vi "spin_diode_effect_test.vi"() -> ()   [LabVIEW 2017]
uses:
  <userlib>/niRF/niQuickSyn/Core/Properties/RF Frequency/PropertyType.ctl
  <userlib>/niRF/niQuickSyn/Core/Properties/RF Power/PropertyType.ctl
  <userlib>/niRF/niQuickSyn/Core/Properties/AM State/PropertyType.ctl
  <userlib>/niRF/niQuickSyn/Core/Properties/FM Sensitivity/PropertyType.ctl
  <userlib>/niRF/niQuickSyn/Core/Properties/VISA Handle/PropertyType.ctl
  <vilib>/Utility/error.llb/DialogType.ctl
  <userlib>/niRF/niQuickSyn/Core/Properties/RF Output/PropertyType.ctl
  <vilib>/DAQmx/write.llb/DAQmx Write (Analog Wfm 1Chan NSamp).vi
  <vilib>/DAQmx/read.llb/DAQmx Read (Analog 1D DBL 1Chan NSamp).vi
  <vilib>/DAQmx/create/channels.llb/DAQmx Create Channel (AO-Voltage-Basic).vi
  <vilib>/DAQmx/configure/timing.llb/DAQmx Timing (Sample Clock).vi
  <vilib>/DAQmx/create/channels.llb/DAQmx Create Channel (AI-Voltage-Basic).vi
  <vilib>/DAQmx/configure/trigger.llb/DAQmx Start Trigger (None).vi
  <vilib>/DAQmx/miscellaneous.llb/DAQmx Fill In Error Info.vi
  <vilib>/Analysis/3filter.llb/Butterworth Filter (DBL).vi
  <userlib>/niRF/niQuickSyn/QuickSyn API.lvlib
  <userlib>/niRF/niQuickSyn/Core/Properties/VISA Handle/VISA Handle.lvclass
  <vilib>/measure/NI_MABase.lvlib
  <userlib>/niRF/niQuickSyn/Core/Properties/RF Output/RF Output.lvclass
  <resource>/objmgr/daqmx.rc
  <vilib>/Analysis/NI_AALBase.lvlib
  <userlib>/niRF/niQuickSyn/Core/Properties/RF Frequency/RF Frequency.lvclass
  <userlib>/niRF/niQuickSyn/Core/Properties/RF Power/RF Power.lvclass
  <userlib>/niRF/niQuickSyn/Core/Properties/AM State/AM State.lvclass
  <userlib>/niRF/niQuickSyn/Core/Properties/FM Sensitivity/FM Sensitivity.lvclass
panel:
  out "SpectrumGraph 3":cluster{dbl[], "data":dbl[]}(graph)
  in  "Number of steps":i32=1000 min=2 step=1
  in  "RF Frequency Stop, Hz":T1=6000000000.0 format="%#_9p"
  out "SpectrumGraph 2":cluster{dbl[], "data":dbl[]}(graph)
  out "Voltage/4":dbl
  in  "AM Depth":T2=100.0 format="%#_9p"
  in  "Amplitude Modulation":T3=enum."Enabled"
  in  "RF Output":bool=TRUE
  in  "error in (no error)":errorcluster
  out "AI.Max":dbl=2.0
  out "AI.Min":dbl=-2.0
  out "AO.Max":dbl=1.0
  out "AO.Min":dbl=-1.0
  out "SpectrumGraph":cluster{dbl[], "data":dbl[]}(graph)
  in  "stop":bool
  out "ms passed":u32=1
  in  "ms to wait":u32=1
  out "error out":errorcluster={"status"=FALSE, "code"=1073676293, "source"="VISA Read in AKIP_read.vi->AKIP_error_check.vi->AKIP_output_on_off.vi->spin_diode_effect_test.vi"}
  in  "AI max":dbl=10.0 format="%0.2f"
  in  "AO max":dbl=0.5 format="%0.2f"
  in  "RF Power, dB":T4=-10.0
  in  "RF Frequency Start, Hz":T1=500000000.0 format="%#_9p"
  in  "Modulation frequency, Hz":dbl=10000.0 format="%0.1p"
  in  "Modulation amplitude, V":dbl=0.5 format="%0.3f"
  in  "AI channel":tag="DAQ6363/ai4"
  in  "AO channel":tag="DAQ6363/ao0"
  in  "Field, Oe":dbl
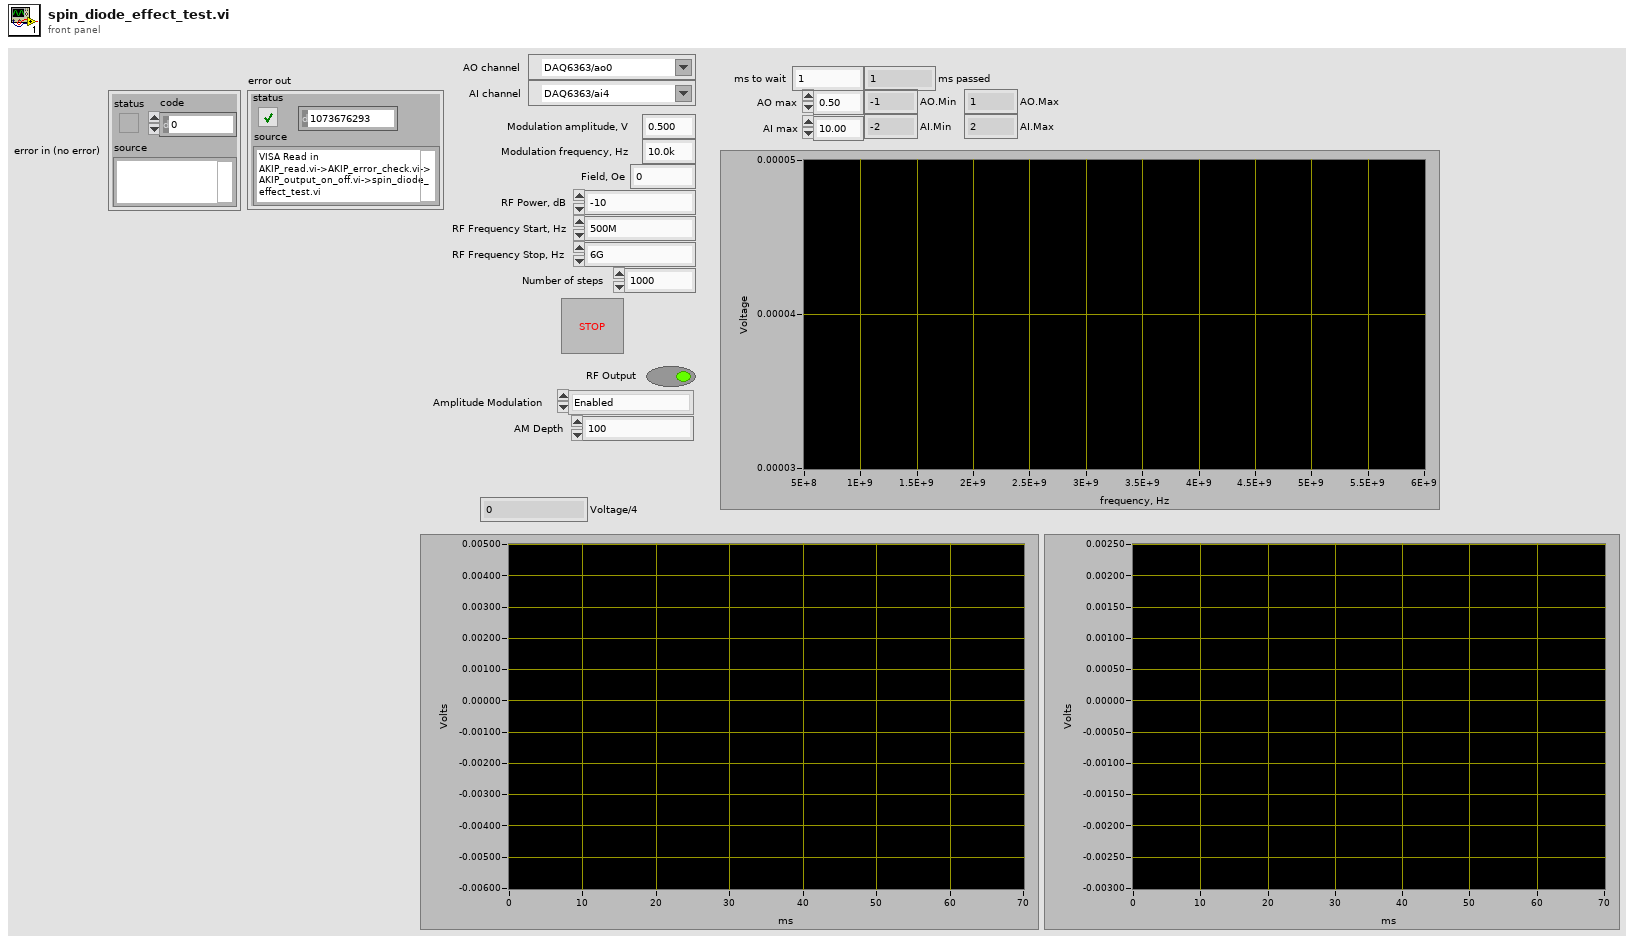
[diagram p1: front panel]
types:
  T1 = typedef "QuickSyn API.lvlib/RF Frequency.lvclass/PropertyType.ctl" = dbl
  T2 = typedef "QuickSyn API.lvlib/FM Sensitivity.lvclass/PropertyType.ctl" = dbl
  T3 = typedef "QuickSyn API.lvlib/AM State.lvclass/PropertyType.ctl" = enum16{"Disabled", "Enabled"}
  T4 = typedef "QuickSyn API.lvlib/RF Power.lvclass/PropertyType.ctl" = dbl
  T5 = enum16{"Sine Wave", "Triangle Wave", "Square Wave", "Sawtooth Wave"}
  T6 = typedef "QuickSyn API.lvlib/RF Output.lvclass/PropertyType.ctl" = bool
  T7 = typedef "DialogType.ctl" = u16
  T8 = typedef "QuickSyn API.lvlib/VISA Handle.lvclass/PropertyType.ctl" = refnum<visa-resource-name>
  T9 = typedef "QuickSyn API.lvlib/QuickSyn.lvclass/Session Handle.ctl" = refnum<data-value>
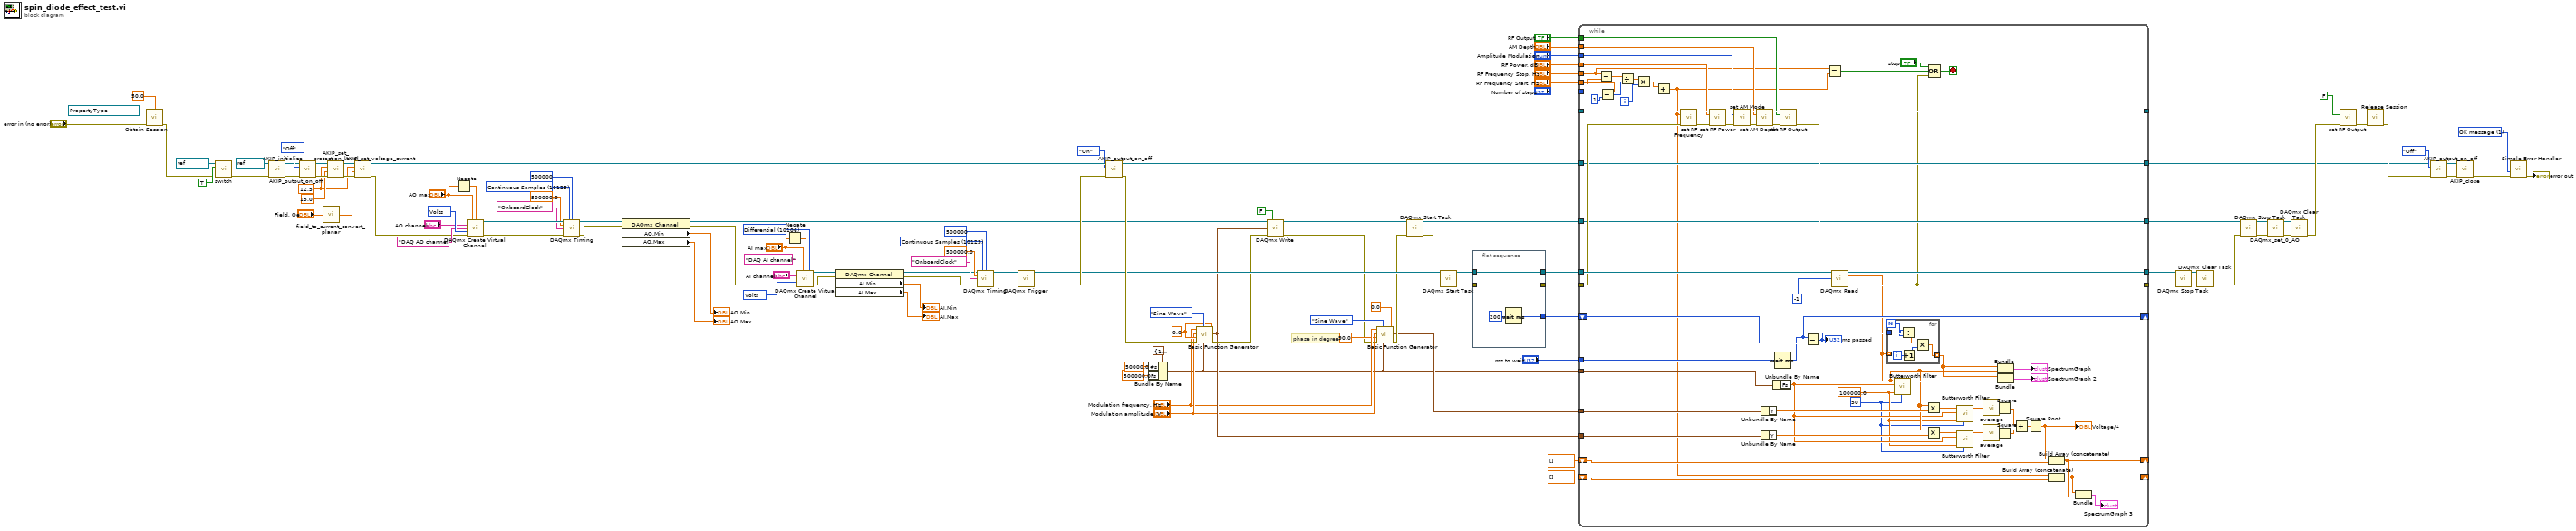
[diagram p0: block diagram]
diagram:
  w38 = 10123 items=["Finite Samples"=10178, "Continuous Samples"=10123, "Hardware Timed Single Point"=12522] ("sample mode")
  w76 = T7 1 items=["no dialog", "OK message", "continue or stop message", "OK message + warnings", "continue/stop + warnings"] ("type of dialog (OK msg:1)")
  w78 = 10348 items=["Volts"=10348, "From Custom Scale"=10065] ("units")
  w79 = 10106 items=["Default"=-1, "RSE"=10083, "NRSE"=10078, "Differential"=10106, "Pseudodifferential"=12529] ("input terminal configuration")
  w89 = 0.0 ("phase")
  w115 = 10123 items=["Finite Samples"=10178, "Continuous Samples"=10123, "Hardware Timed Single Point"=12522] ("sample mode")
  w116 = 10348 items=["Volts"=10348, "From Custom Scale"=10065] ("units")
  w101 = 12.5 ("Voltage")
  # "phase in degrees"
  n1 = call <userlib>:"Obtain Session.vi"("VISA resource name"=T8 "QuickSyn_generator", "Serial Timeout"=50.0, "error in (no error)"="error in (no error)") -> ("Session Handle"=w17:T9, "error out"=w28:errorcluster)  [unwired: 11 in]
  n2 = call "switch.vi"("error in (no error)"=w28, "Positive?"=TRUE, "Switch port (in)"=refnum<visa-resource-name> "Switch") -> ("error out"=w98:errorcluster)  [unwired: 7 in, 1 out]
  n3 = call "AKIP_initialize.vi"("error in (no error)"=w98, "VISA Refnum in"=refnum<visa-resource-name> "AKIP") -> ("error out"=w118:errorcluster, "VISA Refnum out"=w119:refnum<visa-resource-name>)  [unwired: 8 in]
  n4 = call "AKIP_output_on_off.vi"("error in (no error)"=w118, "Enum"=enum16{"On", "Off"}."Off", "VISA Refnum in"=w119) -> ("error out"=w105:errorcluster, "VISA Refnum out"=w104:refnum<visa-resource-name>)  [unwired: 7 in]
  n5 = call "field_to_current_convert_planar.vi"("Field, Oe"="Field, Oe") -> ("Current, A"=w1:dbl)
  n6 = call "AKIP_set_protection_level.vi"("error in (no error)"=w105, "Current Protection Level"=15.0, "Voltage Protection Level"=w101, "VISA resource name (in)"=w104) -> ("error out"=w102:errorcluster, "VISA resource name (out)"=w100:refnum<visa-resource-name>)  [unwired: 6 in]
  n7 = call "AKIP_set_voltage_current.vi"("error in (no error)"=w102, "Current"=w1, "Voltage"=w101, "VISA resource name (in)"=w100) -> ("error out"=w97:errorcluster, "VISA resource name (out)"=w88:refnum<visa-resource-name>)  [unwired: 6 in]
  n8 = Negate(x="AO max") -> (-x=w82:dbl)
  n9 = call-poly <vilib>:"DAQmx Create Virtual Channel.vi"("maximum value"="AO max", "minimum value"=w82, "physical channels"="AO channel", "name to assign"="DAQ AO channel", "units"=w116, "error in"=w97) -> ("task out"=w42:refnum<k21>, "error out"=w41:errorcluster)  [unwired: 8 in]
  n10 = call-poly <vilib>:"DAQmx Timing.vi"("task/channels in"=w42, "sample mode"=w38, "samples per channel"=500000, "rate"=500000.0, "source"=tag "OnboardClock", "error in"=w41) -> ("task out"=w39:refnum<k21>, "error out"=w40:errorcluster)  [unwired: 8 in]
  n11 = property class="DAQmx Channel"(reference=w39, error in=w40) -> (reference out=w65:refnum<k21>, error out=w64:errorcluster, "AO.Min"=→"AO.Min":dbl, "AO.Max"=→"AO.Max":dbl)
  n12 = Negate(x="AI max") -> (-x=w80:dbl)
  n13 = call-poly <vilib>:"DAQmx Create Virtual Channel.vi"("maximum value"="AI max", "minimum value"=w80, "input terminal configuration"=w79, "physical channels"="AI channel", "name to assign"="DAQ AI channel", "units"=w78, "error in"=w64) -> ("task out"=w61:refnum<k21>, "error out"=w59:errorcluster)  [unwired: 7 in]
  n14 = property class="DAQmx Channel"(reference=w61, error in=w59) -> (reference out=w60:refnum<k21>, error out=w58:errorcluster, "AI.Min"=→"AI.Min":dbl, "AI.Max"=→"AI.Max":dbl)
  n15 = call-poly <vilib>:"DAQmx Timing.vi"("task/channels in"=w60, "sample mode"=w115, "samples per channel"=500000, "rate"=500000.0, "source"=tag "OnboardClock", "error in"=w58) -> ("task out"=w113:refnum<k21>, "error out"=w112:errorcluster)  [unwired: 8 in]
  n16 = call-poly <vilib>:"DAQmx Trigger.vi"("task/channels in"=w113, "error in"=w112) -> ("task out"=w55:refnum<k21>, "error out"=w87:errorcluster)  [unwired: 12 in]
  n17 = call "AKIP_output_on_off.vi"("error in (no error)"=w87, "Enum"=enum16{"On", "Off"}."On", "VISA Refnum in"=w88) -> ("error out"=w85:errorcluster, "VISA Refnum out"=w15:refnum<visa-resource-name>)  [unwired: 7 in]
  n18 = Bundle By Name(cluster=cluster{"Fs":dbl, "#s":dbl} {"Fs"=1000.0, "#s"=1000.0} ("sampling info"), "#s"=50000.0, "Fs"=500000.0) -> (w19:cluster{"Fs":dbl, "#s":dbl})
  n19 = call <vilib>:"Basic Function Generator.vi"("offset"=w89, "sampling info"=w19, "signal type"=T5."Sine Wave", "error in (no error)"=w85, "phase"=w89, "amplitude"="Modulation amplitude, V", "frequency"="Modulation frequency, Hz") -> ("error out"=w29:errorcluster, "signal out"=w27:waveform(dbl))  [unwired: 2 in, 1 out]
  n20 = call-poly <vilib>:"DAQmx Write.vi"("task/channels in"=w65, "auto start"=FALSE, "data"=w27, "error in"=w29) -> ("task out"=w84:refnum<k21>, "error out"=w18:errorcluster)  [unwired: 9 in, 1 out]
  n21 = call <vilib>:"Basic Function Generator.vi"("offset"=0.0, "sampling info"=w19, "signal type"=T5."Sine Wave", "error in (no error)"=w18, "phase"=90.0, "amplitude"="Modulation amplitude, V", "frequency"="Modulation frequency, Hz") -> ("error out"=w21:errorcluster, "signal out"=w20:waveform(dbl))  [unwired: 2 in, 1 out]
  n22 = call <vilib>:"DAQmx Start Task.vi"("task/channels in"=w84, "error in"=w21) -> ("task out"=w13:refnum<k21>, "error out"=w54:errorcluster)  [unwired: 12 in]
  n23 = call <vilib>:"DAQmx Start Task.vi"("task/channels in"=w55, "error in"=w54) -> ("task out"=w67:refnum<k21>, "error out"=w66:errorcluster)  [unwired: 12 in]
  n24 = flat-sequence {
    tunnel: w66 -> [w124]
    tunnel: [w124] -> w72
    tunnel: w67 -> [w123]
    tunnel: [w123] -> w73
    tunnel: [w121] -> w69
    frame #0 {
      n25 = Wait (ms)(milliseconds to wait=u32 200) -> (millisecond timer value=w121:u32)
    }
  }
  n26 = while {
    tunnel: w73 -> [w190]
    tunnel: w72 -> [w160]
    tunnel: [w145] -> w71
    tunnel: [w189] -> w70
    shift-right: [w186] -> _
    shift-left: w69 -> [w187]
    tunnel: "ms to wait" -> [w188]
    tunnel: w27 -> [w185]
    tunnel: w20 -> [w184]
    tunnel: w19 -> [w174]
    tunnel: w17 -> [w162]
    tunnel: [w161] -> w16
    tunnel: w15 -> [w158]
    tunnel: [w158] -> w14
    tunnel: w13 -> [w157]
    tunnel: [w157] -> w12
    tunnel: "RF Output" -> [w156]
    tunnel: "AM Depth" -> [w155]
    tunnel: "Amplitude Modulation" -> [w154]
    tunnel: "RF Power, dB" -> [w153]
    tunnel: "Number of steps" -> [w151]
    tunnel: "RF Frequency Stop, Hz" -> [w142]
    tunnel: "RF Frequency Start, Hz" -> [w144]
    shift-right: [w137] -> _
    shift-left: dbl[] [] -> [w138]
    shift-right: [w134] -> _
    shift-left: T1[] [] -> [w135]
    i -> [w147]
    stop <- w140 stop-if-true
    w126 = 100000.0 ("low cutoff freq: fl")
    w125 = 50 ("order")
    n27 = Subtract(x=w142, y=w144) -> (x-y=w152:T1)
    n28 = Subtract(x=w151, y=1) -> (x-y=w149:i32)
    n29 = Divide(x=w152, y=w149) -> (x/y=w148:T1)
    n30 = Multiply(x=w148, y=w147) -> (x*y=w143:T1)
    n31 = Add(x=w143, y=w144) -> (x+y=w136:T1)
    n32 = call <userlib>:"set RF Frequency.vi"("Session Handle in"=w162, "RF Frequency, Hz (200M)"=w136, "error in (no error)"=w160) -> ("Session Handle out"=w165:T9, "error out"=w166:errorcluster)  [unwired: 11 in]
    n33 = call <userlib>:"set RF Power.vi"("Session Handle in"=w165, "RF Power, dB (0)"=w153, "error in (no error)"=w166) -> ("Session Handle out"=w168:T9, "error out"=w167:errorcluster)  [unwired: 11 in]
    n34 = call <userlib>:"set AM Mode.vi"("Session Handle in"=w168, "AM State"=w154, "error in (no error)"=w167) -> ("Session Handle out"=w163:T9, "error out"=w164:errorcluster)  [unwired: 11 in]
    n35 = call <userlib>:"set AM Depth.vi"("Session Handle in"=w163, "AM Depth"=w155, "error in (no error)"=w164) -> ("Session Handle out"=w169:T9, "error out"=w170:errorcluster)  [unwired: 11 in]
    n36 = Unbundle By Name(w184) -> ("Y"=w176:dbl[])
    n37 = Unbundle By Name(w185) -> ("Y"=w177:dbl[])
    n38 = Unbundle By Name(w174) -> ("Fs"=w127:dbl)
    n39 = Wait (ms)(milliseconds to wait=w188) -> (millisecond timer value=w186:u32)
    n40 = call <userlib>:"set RF Output.vi"("Session Handle in"=w169, "RF Output (False)"=w156, "error in (no error)"=w170) -> ("Session Handle out"=w161:T9, "error out"=w159:errorcluster)  [unwired: 11 in]
    n41 = Subtract(x=w186, y=w187) -> (x-y=w178:u32)
    "ms passed" <- w178
    n42 = Equal?(x=w142, y=w136) -> (x = y?=w141:bool)
    n43 = call-poly <vilib>:"DAQmx Read.vi"("task/channels in"=w190, "number of samples per channel"=-1, "error in"=w159) -> ("task out"=w189:refnum<k21>, "data"=w132:dbl[], "error out"=w145:errorcluster)  [unwired: 10 in]
    n44 = for {
      N -> [w195]
      tunnel: [w192] -> w172 mode=indexing
      tunnel: w132 -> [_] mode=indexing
      tunnel: w178 -> [w196]
      i -> [w197]
      n45 = Divide(x=w196, y=w195) -> (x/y=w194:dbl)
      n46 = Increment(x=w197) -> (x+1=w193:i32)
      n47 = Multiply(x=w194, y=w193) -> (x*y=w192:dbl)
    }
    n48 = call-poly <vilib>:"Butterworth Filter.vi"("order"=w125, "low cutoff freq: fl"=w126, "sampling freq: fs"=w127, "X"=w132) -> ("Filtered X"=w171:dbl[])  [unwired: 4 in, 1 out]
    n49 = Multiply(x=w132, y=w176) -> (x*y=w131:dbl[])
    n50 = Multiply(x=w132, y=w177) -> (x*y=w129:dbl[])
    n51 = Compound Arithmetic op=OR("stop", w141, w145) -> (w140:bool)
    n52 = call-poly <vilib>:"Butterworth Filter.vi"("order"=w125, "low cutoff freq: fl"=w126, "sampling freq: fs"=w127, "X"=w131) -> ("Filtered X"=w130:dbl[])  [unwired: 4 in, 1 out]
    n53 = call-poly <vilib>:"Butterworth Filter.vi"("order"=w125, "low cutoff freq: fl"=w126, "sampling freq: fs"=w127, "X"=w129) -> ("Filtered X"=w128:dbl[])  [unwired: 4 in, 1 out]
    n54 = call "average.vi"("Array"=w130) -> ("Average"=w183:dbl)
    n55 = call "average.vi"("Array"=w128) -> ("Average"=w182:dbl)
    n56 = Square(x=w183) -> (x^2=w181:dbl)
    n57 = Square(x=w182) -> (x^2=w180:dbl)
    n58 = Bundle(w172, "data"=w132) -> (→"SpectrumGraph":cluster{dbl[], "data":dbl[]})  [unwired: 1 in]
    n59 = Bundle(w172, "Filtered X"=w171) -> (→"SpectrumGraph 2":cluster{dbl[], "Filtered X":dbl[]})  [unwired: 1 in]
    n60 = Add(x=w181, y=w180) -> (x+y=w179:dbl)
    n61 = Square Root(x=w179) -> (sqrt(x)=w139:dbl)
    "Voltage/4" <- w139
    n62 = Build Array (concatenate)(w139, w138) -> (w137:dbl[])
    n63 = Build Array (concatenate)(w136, w135) -> (w134:T1[])
    n64 = Bundle(w134, w137) -> (→"SpectrumGraph 3":cluster{T1[], dbl[]})  [unwired: 1 in]
  }
  n65 = call <vilib>:"DAQmx Stop Task.vi"("task/channels in"=w70, "error in"=w71) -> ("task out"=w74:refnum<k21>, "error out"=w75:errorcluster)  [unwired: 12 in]
  n66 = call <vilib>:"DAQmx Clear Task.vi"("task in"=w74, "error in"=w75) -> ("error out"=w34:errorcluster)  [unwired: 13 in]
  n67 = call <vilib>:"DAQmx Stop Task.vi"("task/channels in"=w12, "error in"=w34) -> ("task out"=w33:refnum<k21>, "error out"=w32:errorcluster)  [unwired: 12 in]
  n68 = call "DAQmx_set_0_AO.vi"("Refnum in"=w33, "error in (no error)"=w32) -> ("Refnum out"=w31:refnum<k21>, "error out"=w30:errorcluster)  [unwired: 12 in]
  n69 = call <vilib>:"DAQmx Clear Task.vi"("task in"=w31, "error in"=w30) -> ("error out"=w51:errorcluster)  [unwired: 13 in]
  n70 = call <userlib>:"set RF Output.vi"("Session Handle in"=w16, "RF Output (False)"=T6 FALSE, "error in (no error)"=w51) -> ("Session Handle out"=w50:T9, "error out"=w49:errorcluster)  [unwired: 11 in]
  n71 = call <userlib>:"Release Session.vi"("Session Handle"=w50, "error in (no error)"=w49) -> ("error out"=w46:errorcluster)  [unwired: 13 in]
  n72 = call "AKIP_output_on_off.vi"("error in (no error)"=w46, "Enum"=enum16{"On", "Off"}."Off", "VISA Refnum in"=w14) -> ("error out"=w48:errorcluster, "VISA Refnum out"=w47:refnum<visa-resource-name>)  [unwired: 7 in]
  n73 = call "AKIP_close.vi"("error in (no error)"=w48, "VISA Refnum in"=w47) -> ("error out"=w45:errorcluster)  [unwired: 8 in, 1 out]
  n74 = call <vilib>:"Simple Error Handler.vi"("type of dialog (OK msg:1)"=w76, "error in (no error)"=w45) -> ("error out"=→"error out":errorcluster)  [unwired: 3 in, 4 out]
